vi "Sensor_geradeaus_links.vi"() -> (3 "Distanz Array":dbl)   [LabVIEW 2016]
doc: "SubVI liest IR Sensor aus und berechnet Servo-Wert anhand der erstellten Kurve\n05.04.17_Tloe"
uses:
  <vilib>/myRIO/Instrument Drivers/Onboard IO/AI/typedefs/AI Reference.ctl
  <vilib>/myRIO/Common/Instrument Driver Framework/Utilities/typedefs/myRIO Generic Hardware Reference.ctl
  <vilib>/myRIO/Common/Instrument Driver Framework/Utilities/typedefs/Hardware Version Enum.ctl
  <vilib>/myRIO/Common/Instrument Driver Framework/Utilities/typedefs/myRIO v1.0 Reference.ctl
  <vilib>/myRIO/Common/Instrument Driver Framework/Utilities/typedefs/Generic FPGA Reference.ctl
  <vilib>/myRIO/Common/Instrument Driver Framework/myRIO v1.0/AI/typedefs/AI Channels List.ctl
  <vilib>/myRIO/Common/Instrument Driver Framework/myRIO v1.0/AI/typedefs/AI Channels Enum.ctl
  <vilib>/myRIO/Common/Instrument Driver Framework/Utilities/typedefs/Analog Scaling Constants List.ctl
  <vilib>/myRIO/Common/Instrument Driver Framework/Utilities/typedefs/Analog Scaling Constants.ctl
  <vilib>/userdefined/High Color/nirio_resource_hc.ctl
  <vilib>/myRIO/Instrument Drivers/Onboard IO/AI/vis/Read.vi
  <vilib>/myRIO/Common/Instrument Driver Framework/myRIO v1.0/AI/vis/myRIO v1.1 Open AI.vi
  <vilib>/myRIO/Common/Instrument Driver Framework/Utilities/vis/Is FPGA Ref Available.vi
  <vilib>/myRIO/Common/Instrument Driver Framework/Utilities/vis/Validate Channels.vi
  <vilib>/myRIO/Common/Instrument Driver Framework/myRIO v1.0/AI/vis/myRIO v1.0 Reserve AI.vi
  <vilib>/myRIO/Common/Instrument Driver Framework/myRIO v1.0/AI/vis/myRIO v1.0 Build MUX Configuration AI.vi
  <vilib>/myRIO/Common/Instrument Driver Framework/myRIO v1.0/Resource Manager/vis/myRIO v1.0 Reserve Channel List.vi
  <vilib>/myRIO/Common/Instrument Driver Framework/myRIO v1.0/Resource Manager/vis/myRIO v1.0 Reserve Channel.vi
  <vilib>/myRIO/Common/Instrument Driver Framework/myRIO v1.0/Resource Manager/vis/myRIO v1.0 Unreserve Channel.vi
  <vilib>/myRIO/Common/Instrument Driver Framework/myRIO v1.0/Resource Manager/vis/myRIO v1.0 Build Mutex Name.vi
  <vilib>/myRIO/Common/Instrument Driver Framework/myRIO v1.0/AI/vis/myRIO v1.0 Read AI.vi
  <vilib>/Utility/error.llb/Error Cluster From Error Code.vi
  <vilib>/myRIO/Common/Instrument Driver Framework/myRIO v1.0/myRIO v1.0 Close.vi
  <vilib>/myRIO/Common/Instrument Driver Framework/Utilities/vis/IO Manager.vi
  <vilib>/myRIO/Common/Instrument Driver Framework/Utilities/vis/Configuration Manager.vi
  <vilib>/myRIO/Common/Instrument Driver Framework/myRIO v1.0/AI/vis/myRIO v1.0 Get Scaling Constants AI.vi
  <vilib>/myRIO/Common/Instrument Driver Framework/myRIO v1.0/myRIO v1.1 Open.vi
  <vilib>/Utility/VariantDataType/GetNumericInfo.vi
  <vilib>/myRIO/Instrument Drivers/Onboard IO/AI/vis/myRIO AI Open.xnode
  <vilib>/myRIO/Express VI/Onboard IO/AI/AI Express VI.xnode
  <vilib>/myRIO/Instrument Drivers/Onboard IO/AI/AI.lvlib
  <vilib>/ptbypt/NI_PtbyPt.lvlib
panel:
  in  "Distanzen IR Sensor":dbl[](array[numeric])=[10.0, 15.0, 20.0, 25.0, 30.0, 35.0, 40.0, 45.0, 50.0, 60.0, 70.0, 80.0, 90.0, 100.0, 110.0, 120.0, 130.0, 140.0, 150.0]
  in  "Messwerte IR Sensor vorne rechts":dbl[](array[numeric])=[3.491, 2.5228, 1.9988, 1.6937, 1.489, 1.3496, 1.2344, 1.1528, 1.0856, 0.971, 0.881, 0.782, 0.68, 0.598, 0.538, 0.483, 0.435, 0.395, 0.362]
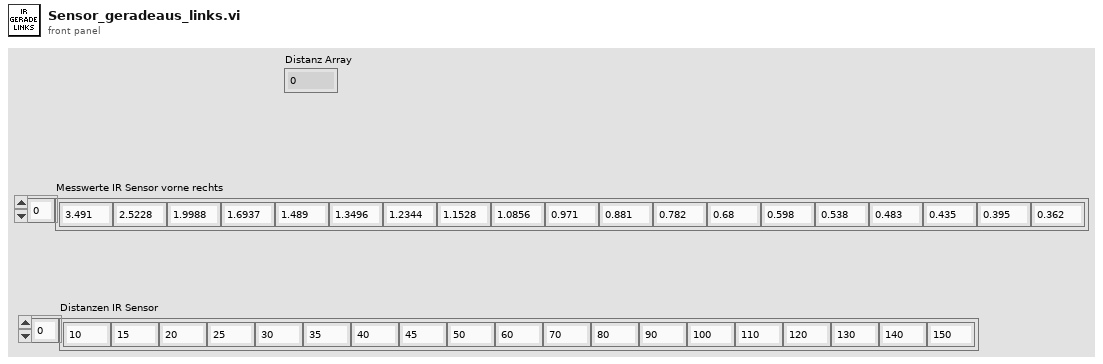
[diagram p1: front panel]
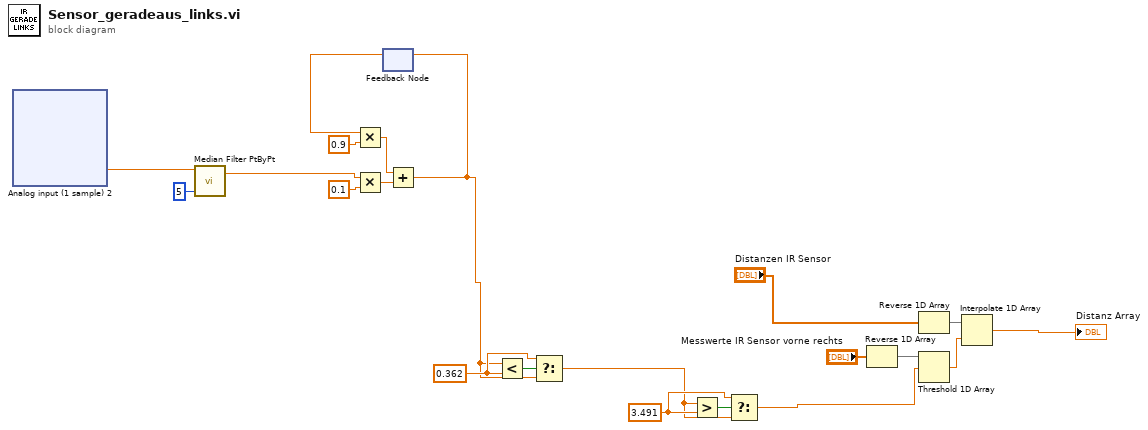
[diagram p0: block diagram]
diagram:
  w7 = 3.491 ("y")
  w9 = 0.362 ("y")
  n1 = xnode "Analog input (1 sample) 2"() -> ("A/AI0 (Pin 3)"=w2:dbl)  [unwired: 1 in, 1 out]
  n2 = call <vilib>:"Median Filter PtByPt.vi"("rank"=5, "x"=w2) -> ("Filtered x"=w16:dbl)  [unwired: 2 in, 1 out]
  n3 = Multiply(x=w16, y=0.1) -> (x*y=w19:dbl)
  n4 = feedback #1() -> (w17:dbl)  [unwired: 1 in]
  n5 = Multiply(x=w17, y=0.9) -> (x*y=w18:dbl)
  n6 = Add(x=w18, y=w19) -> (x+y=w3:dbl)
  n7 = feedback-in #1(w3) -> ()
  n8 = Less?(x=w3, y=w9) -> (x < y?=w10:bool)
  n9 = Select(t=w9, s=w10, f=w3) -> (s? t:f=w6:dbl)
  n10 = Greater?(x=w6, y=w7) -> (0:w8:bool)
  n11 = Select(t=w7, s=w8, f=w6) -> (s? t:f=w5:dbl)
  n12 = Reverse 1D Array(array="Messwerte IR Sensor vorne rechts") -> (reversed array=w12:dbl[])
  n13 = Reverse 1D Array(array="Distanzen IR Sensor") -> (reversed array=w11:dbl[])
  n14 = Threshold 1D Array(2:w5, 3:w12) -> (0:w15:dbl)  [unwired: 1 in]
  n15 = Interpolate 1D Array(1:w15, 2:w11) -> (0:→"Distanz Array":dbl)
